vi "VciEnumDeviceClose.vi"(3 "error in":errorcluster {"code" format="%.0x"}, 5 "Enum Handle in":u32) -> (0 "error out":errorcluster {"code" format="%.0x"})   [LabVIEW 2011]
doc: "Closes the specified device enumeration handle."
uses:
  vcilva.dll
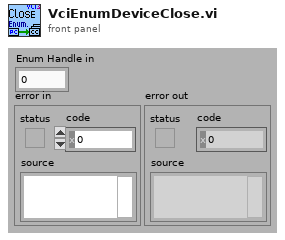
[diagram p1: front panel]
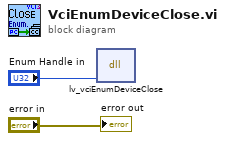
[diagram p0: block diagram]
diagram:
  n1 = dll-call lib="vcilva.dll" fn="lv_vciEnumDeviceClose"("hEnum"="Enum Handle in") -> ()  [unwired: 5 in, 2 out]
  "error out" <- "error in"
